vi "FPGA_DIOReadDO_PWMDutyCycle.vi"(8 "error in (no error)":errorcluster, 9 "DO_PWM Index":i8, 11 "DIODeviceRef":T1) -> (0 "error out":errorcluster, 2 "DO_PWMDutyCycle":u8, 3 "DIODeviceRef":T1)   [LabVIEW 2017]
uses:
  <vilib>/Rock Robotics/SystemInterfaces/DIO/FPGA_DIODevRef.ctl
  <vilib>/Rock Robotics/SystemInterfaces/System/FPGA_SystemFPGA Ref Global.vi
  <vilib>/Utility/error.llb/Error Cluster From Error Code.vi
  <vilib>/rvi/errors/niLvFpgaAdjustHostInterfaceError.vi
  <vilib>/rvi/interface/nirviReadWriteControl/nirviReadWriteControl.xnode
  <vilib>/Rock Robotics/SystemInterfaces/System/FPGA_SystemFRC FPGA Ref.ctl
  <vilib>/rvi/interface/Simulation/niFpgaSimulationCallBeginRW.vi
  NiFpgaLv.dll
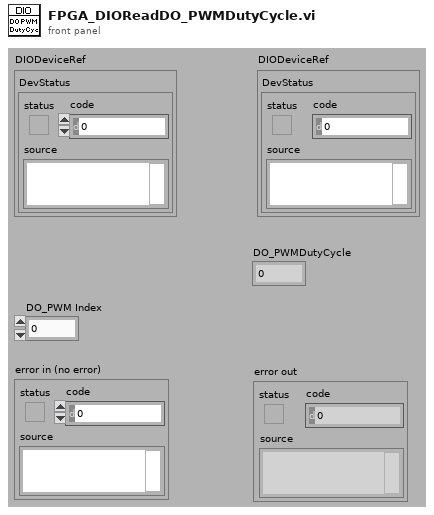
[diagram p1: front panel]
types:
  T1 = typedef "FPGA_DIODevRef.ctl" = cluster{"DevStatus":errorcluster}
  T2 = typedef "FPGA_SystemFRC FPGA Ref.ctl" = refnum<k20>
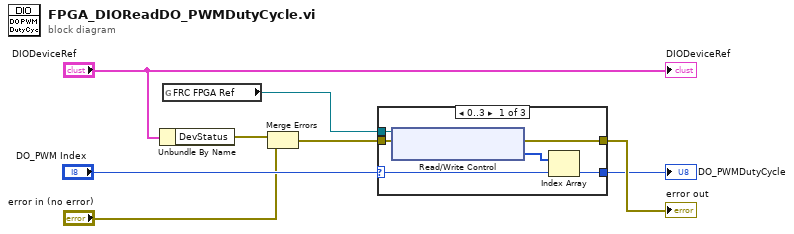
[diagram p0: block diagram]
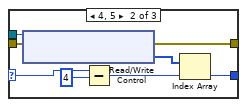
[diagram p2: hidden frame]
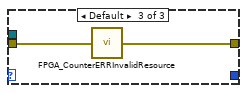
[diagram p3: hidden frame]
diagram:
  n1 = Unbundle By Name("DIODeviceRef") -> ("DevStatus"=w5:errorcluster)
  n2 = global read "FPGA_SystemFPGA Ref Global.vi" "FRC FPGA Ref"() -> (w6:T2)
  n3 = Merge Errors(w5, "error in (no error)") -> (w4:errorcluster)
  n4 = case shown="0..3" "DO_PWM Index" {
    selector: "DO_PWM Index" -> [w10 w18 _]
    tunnel: [w14 w22 w23] -> w8
    tunnel: w6 -> [w12 w20 _]
    tunnel: w4 -> [w11 w19 w24]
    tunnel: [w9 w15 _] -> w1
    frame 0..3 {
      n5 = xnode "Read/Write Control"("FPGA VI Reference In"=w12, "error in"=w11) -> ("error out"=w14:errorcluster, "DIO.PWMDutyCycleA"=w13:u8[])  [unwired: 1 out]
      n6 = Index Array(array=w13, index=w10) -> (element=w9:u8)
    }
    frame 4, 5 {
      n7 = xnode "Read/Write Control"("FPGA VI Reference In"=w20, "error in"=w19) -> ("error out"=w22:errorcluster, "DIO.PWMDutyCycleB"=w21:u8[])  [unwired: 1 out]
      n8 = Subtract(x=w18, y=i8 4 ("x")) -> (x-y=w17:i8)
      n9 = Index Array(array=w21, index=w17) -> (element=w15:u8)
    }
    frame Default {
      n10 = call <vilib>:"FPGA_CounterERRInvalidResource.vi"("error in (no error)"=w24) -> ("error out"=w23:errorcluster)
    }
  }
  "DO_PWMDutyCycle" <- w1
  "error out" <- w8
  "DIODeviceRef" <- "DIODeviceRef"
